vi "Check Entry State.vi"(8 "error in (no error)":refnum<class "MultiErrors.lvclass">, 11 "Sequence Validation in":refnum<class "Sequence Validation.lvclass">) -> (0 "error out":refnum<class "MultiErrors.lvclass">, 3 "Sequence Validation out":refnum<class "Sequence Validation.lvclass">)   [LabVIEW 2020, in "VolatusSeq.lvlib" / "Sequence Validation.lvclass"]
uses:
  Sequence Validation.lvclass
  Sequence Validation.lvclass/Sequence Validation.ctl
  Sequence Config/Sequence Config.lvclass
  VolatusErrorUtilities/MultiErrors/MultiErrors.lvclass
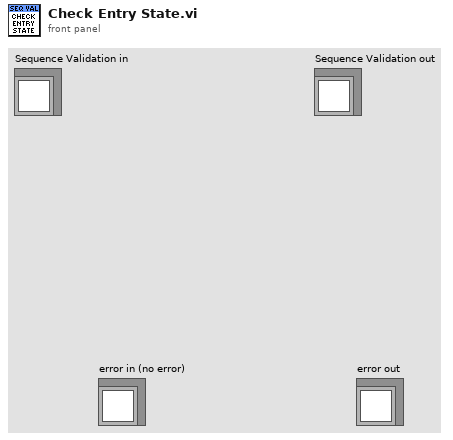
[diagram p1: front panel]
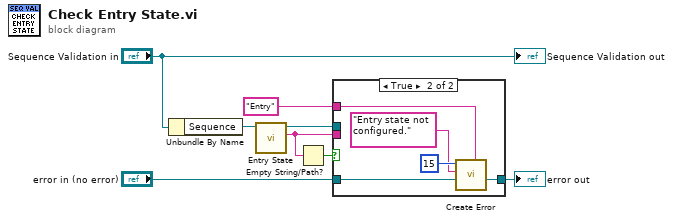
[diagram p0: block diagram]
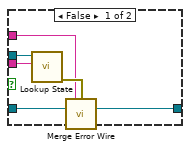
[diagram p2: hidden frame]
diagram:
  n1 = Unbundle By Name("Sequence Validation in") -> ("Sequence"=w7:refnum<class "Sequence Config.lvclass">)
  n2 = call "Entry State.vi"("Sequence Config in"=w7) -> ("Entry State"=w5:string, "Sequence Config out"=w4:refnum<class "Sequence Config.lvclass">)  [unwired: 9 in]
  n3 = Empty String/Path?(string/path=w5) -> (empty?=w6:bool)
  n4 = case shown="True" w6 {
    tunnel: w5 -> [w9 _]
    tunnel: w4 -> [w10 _]
    tunnel: "error in (no error)" -> [w12 w19]
    tunnel: [w11 w17] -> w2
    tunnel: "Entry" ("Context") -> [w13 w16]
    frame False {
      n5 = call "Lookup State.vi"("State"=w9, "Sequence Config in"=w10) -> ("error out"=w14:errorcluster)  [unwired: 7 in, 2 out]
      n6 = call "Merge Error Wire.vi"("Local Context (None)"=w13, "error in (no error)"=w14, "MultiErrors in"=w12) -> ("MultiErrors out"=w11:refnum<class "MultiErrors.lvclass">)  [unwired: 12 in]
    }
    frame True {
      n7 = call "Create Error.vi"("Local Context (None)"=w16, "MultiErrors in"=w19, "Message"="Entry state not configured.", "Code"=15) -> ("MultiErrors out"=w17:refnum<class "MultiErrors.lvclass">)  [unwired: 7 in]
    }
  }
  "error out" <- w2
  "Sequence Validation out" <- "Sequence Validation in"
